vi "TCP- Server.vi"() -> ()   [LabVIEW 2015]
doc: "Demonstrates how to use network streams to pass data and commands between two running VIs. It displays waveform data that is received from the target VI and sends commands to update the frequency of the generated signal."
uses:
  support/Network Stream Global Stop.vi
panel:
  in  "Cluster":cluster{"Frequency":i32}={"Frequency"=10}
  in  "Server Closed":string="The server VI closed the connection."
  out "value":T1
  in  "Client Closed":string="The client VI closed the connection."
  in  "Frequency":i32=10
  in  "Stop":bool
  # "Overview: Demonstrates how to use Network Streams to pass data and commands between two running VIs.\nRequirements: Windows\nInstructions:\n1. Make sure Simple Network Streams - Target.vi is already running.\n2. Run this VI.\n3. Change the Frequency value and observe the change in data that results from sending the new frequency value to the Target VI.\n4. Change the Read Speed value in this VI, and the Write Speed value in the Target VI, and observe the resulting values of Available Elements to Read and Available Elements to Write.\n5. Click Stop to stop the VI."
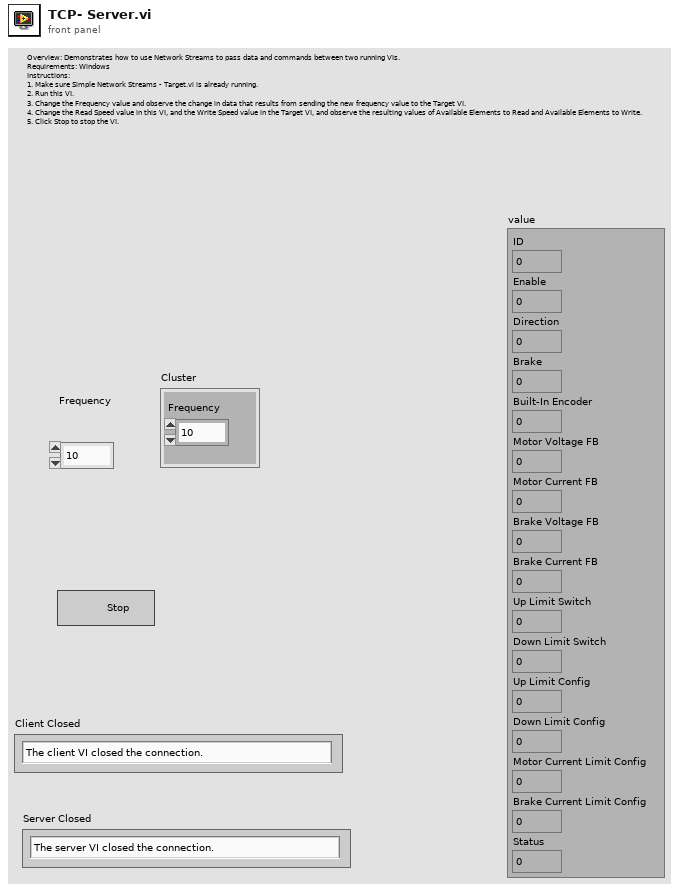
[diagram p1: front panel]
types:
  T1 = cluster{"ID":dbl, "Enable":dbl, "Direction":dbl, "Brake":dbl, "Built-In Encoder":dbl, "Motor Voltage FB":dbl, "Motor Current FB":dbl, "Brake Voltage FB":dbl, "Brake Current FB":dbl, "Up Limit Switch":dbl, "Down Limit Switch":dbl, "Up Limit Config":dbl, "Down Limit Config":dbl, "Motor Current Limit Config":dbl, "Brake Current Limit Config":dbl, "Status":dbl}
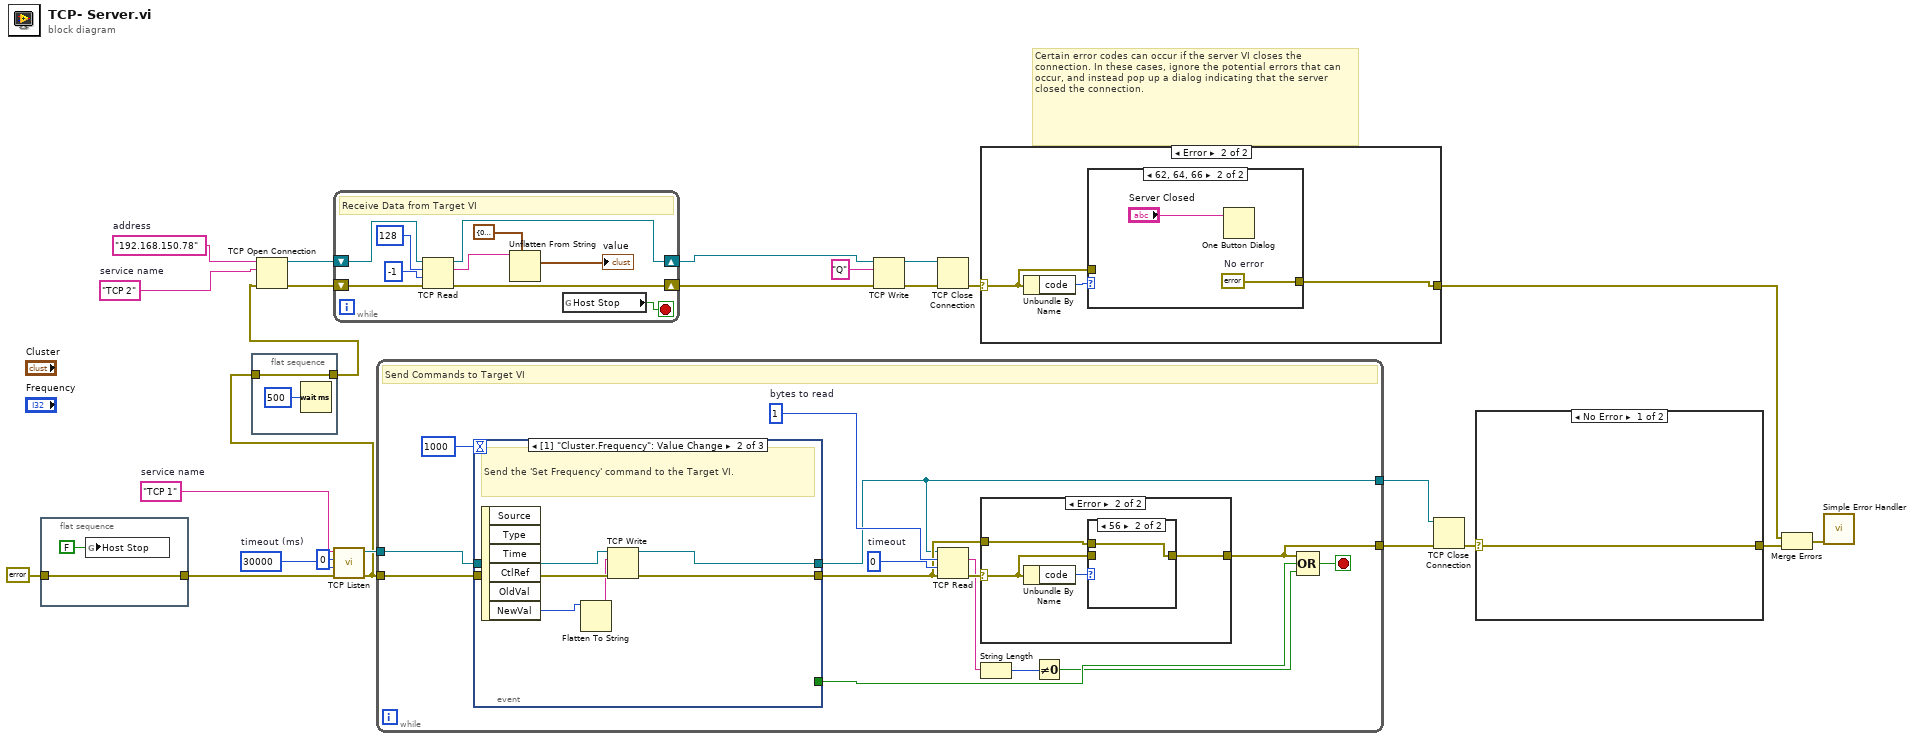
[diagram p0: block diagram]
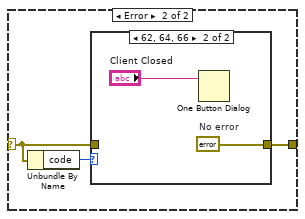
[diagram p4: hidden frame]
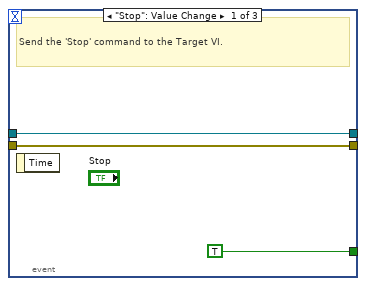
[diagram p8: hidden frame]
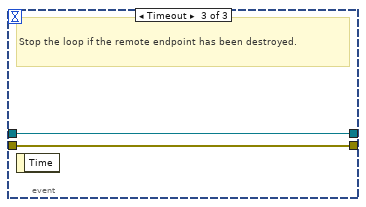
[diagram p9: hidden frame]
diagram:
  w4 = "TCP 2"  # service name
  w17 = "192.168.150.78"  # address
  w23 = "TCP 1"  # service name
  w22 = 30000  # timeout (ms)
  # "Certain error codes can occur if the server VI closes the connection. In these cases, ignore the potential errors that can occur, and instead pop up a dialog indicating that the server closed the connection."
  n1 = flat-sequence {
    tunnel: errorcluster {"status"=FALSE, "code"=0, "source"=""} ("error out") -> [w25]
    tunnel: [w25] -> w13
    frame #0 {
      n2 = global write "Network Stream Global Stop.vi" "Host Stop"(FALSE ("Host Stop")) -> ()
    }
  }
  n3 = flat-sequence {
    tunnel: w1 -> [w27]
    tunnel: [w27] -> w2
    frame #0 {
      n4 = Wait (ms)(milliseconds to wait=u32 500) -> ()  [unwired: 1 out]
    }
  }
  n5 = TCP Open Connection(address=w17, remote port or service name=w4, error in (no error)=w2) -> (connection ID=w15:refnum<k5>, error out=w16:errorcluster)  [unwired: 2 in]
  n6 = while "Target->Host Data Reader" {
    shift-right: [w31] -> w8
    shift-left: w16 -> [w32]
    shift-right: [w30] -> w7
    shift-left: w15 -> [w29]
    stop <- w38 stop-if-true
    # "Receive Data from Target VI"
    n7 = TCP Read(connection ID=w29, bytes to read=128, error in (no error)=w32, 9:-1 ("timeout ms (25000)")) -> (connection ID out=w30:refnum<k5>, data out=w35:string, error out=w31:errorcluster)  [unwired: 1 in]
    n8 = Unflatten From String(type=T1 {"ID"=0.0, "Enable"=0.0, "Direction"=0.0, "Brake"=0.0, "Built-In Encoder"=0.0, "Motor Voltage FB"=0.0, "Motor Current FB"=0.0, "Brake Voltage FB"=0.0, "Brake Current FB"=0.0, "Up Limit Switch"=0.0, "Down Limit Switch"=0.0, "Up Limit Config"=0.0, "Down Limit Config"=0.0, "Motor Current Limit Config"=0.0, "Brake Current Limit Config"=0.0, "Status"=0.0} ("MirrorCoverMotor"), binary string=w35) -> (value=→"value":T1)  [unwired: 3 in, 2 out]
    n9 = global read "Network Stream Global Stop.vi" "Host Stop"() -> (w38:bool)
  }
  n10 = call <vilib>:"TCP Listen.vi"("error in (no error)"=w13, "timeout ms (wait forever: -1)"=w22, "port"=u16 0, "service name"=w23) -> ("error out"=w1:errorcluster, "connection ID"=w21:refnum<k5>)  [unwired: 3 in, 3 out]
  n11 = while "Host->Target Command Writer" {
    tunnel: w1 -> [w51]
    tunnel: w21 -> [w50]
    tunnel: [w40] -> w19
    tunnel: [w39] -> w18
    stop <- w43 stop-if-true
    w46 = 0  # timeout
    w45 = 1  # bytes to read
    # "Send Commands to Target VI"
    n12 = event shown="[1] \"Cluster.Frequency\": Value Change" {
      selector: _ -> [_ _ _]
      dyn-events: _ -> [_ _ _]
      timeout: 1000 -> [_ _ _]
      tunnel: [TRUE _ _] -> w42
      tunnel: w51 -> [w61 w68 w69]
      tunnel: w50 -> [w60 w67 w70]
      tunnel: [w61 w66 w69] -> w44
      tunnel: [w60 w65 w70] -> w39
      event "Stop": Value Change {
        # "Send the 'Stop' command to the Target VI."
        n13 = event-data() -> ()  [unwired: 2 out]
      }
      event "Cluster.Frequency": Value Change {
        # "Send the 'Set Frequency' command to the Target VI."
        n14 = event-data() -> ("NewVal"=w64:i32)  [unwired: 6 out]
        n15 = Flatten To String(anything=w64) -> (data string=w63:string)  [unwired: 3 in, 2 out]
        n16 = TCP Write(connection ID=w67, data in=w63, error in (no error)=w68) -> (connection ID out=w65:refnum<k5>, error out=w66:errorcluster)  [unwired: 2 out]
      }
      event Timeout {
        # "Stop the loop if the remote endpoint has been destroyed."
        n17 = event-data() -> ()  [unwired: 2 out]
      }
    }
    n18 = TCP Read(connection ID=w39, bytes to read=w45, error in (no error)=w44, 9:w46) -> (data out=w48:string, error out=w49:errorcluster)  [unwired: 2 out]
    n19 = case shown="Error" w49 {
      selector: w49 -> [w53 w56]
      tunnel: [w53 w54] -> w40
      tunnel: w44 -> [_ w55]
      frame No Error {
      }
      frame Error {
        n20 = Unbundle By Name(w56) -> ("code"=w57:i32)
        n21 = case shown="56" w57 {
          tunnel: w56 -> [w58 _]
          tunnel: w55 -> [_ w59]
          tunnel: [w58 w59] -> w54
          frame Default {
          }
          frame 56 {
          }
        }
      }
    }
    n22 = String Length(string=w48) -> (length=w47:i32)
    n23 = Not Equal To 0?(x=w47) -> (x != 0?=w41:bool)
    n24 = Compound Arithmetic op=OR(w40, w42, w41) -> (w43:bool)
  }
  n25 = TCP Write(connection ID=w7, data in="Q", error in (no error)=w8) -> (connection ID out=w9:refnum<k5>, error out=w10:errorcluster)  [unwired: 2 out]
  n26 = TCP Close Connection(connection ID=w9, error in (no error)=w10) -> (error out=w12:errorcluster)  [unwired: 1 in, 1 out]
  n27 = case shown="Error" w12 {
    selector: w12 -> [w71 w73]
    tunnel: [w71 w72] -> w6
    frame No Error {
    }
    frame Error {
      n28 = Unbundle By Name(w73) -> ("code"=w74:i32)
      n29 = case shown="62, 64, 66" w74 {
        tunnel: w73 -> [w75 _]
        tunnel: [w75 w77] -> w72
        frame Default {
        }
        frame 62, 64, 66 {
          w77 = errorcluster {"status"=FALSE, "code"=0, "source"=""}  # No error
          n30 = One Button Dialog(message="Server Closed") -> ()  [unwired: 1 in, 1 out]
        }
      }
    }
  }
  n31 = TCP Close Connection(connection ID=w18, error in (no error)=w19) -> (error out=w20:errorcluster)  [unwired: 2 out]
  n32 = case shown="No Error" w20 {
    selector: w20 -> [w78 w80]
    tunnel: [w78 w79] -> w5
    frame No Error {
    }
    frame Error {
      n33 = Unbundle By Name(w80) -> ("code"=w81:i32)
      n34 = case shown="62, 64, 66" w81 {
        tunnel: w80 -> [w82 _]
        tunnel: [w82 w84] -> w79
        frame Default {
        }
        frame 62, 64, 66 {
          w84 = errorcluster {"status"=FALSE, "code"=0, "source"=""}  # No error
          n35 = One Button Dialog(message="Client Closed") -> ()  [unwired: 1 in, 1 out]
        }
      }
    }
  }
  n36 = Merge Errors(w6, w5) -> (w24:errorcluster)
  n37 = call <vilib>:"Simple Error Handler.vi"("error in (no error)"=w24) -> ()  [unwired: 4 in, 5 out]
